vi "Side E.vi"(0 "Input Image":T7, 1 "Calibrated Image":T7, 5 "Ref ROI Parameters":T6={"Ref Line ROI Before Transformation"={"Global Rectangle"=[], "Contours"=[]}, "Ref ROI Search Direction"=2, "Ref ROI Edge Options"={"Edge Polarity"=2, "Kernel Size"=3, "Width"=3, "Minimum Edge Strength"=50.0, "Interpolation Type"=enum."Zero Order", "Data Processing Method"=enum."Average"}, "Ref ROI Line Options"={"Number of Lines"=1, "Type"=enum."Best Edge Rake", "Min. Score"=10.0, "Max. Score"=1000.0, "Orientation"=0.0, "Angle Range"=10.0, "Angle Tolerance"=10.0, "Step Size"=14, "Min. SNR (db)"=0.0, "Min. Points (%)"=25.0, "Hough Iterations"=5}, "Ref ROI Overlay"=FALSE, "Ref Rake Line Overlay 2"=FALSE, "Ref Edge/Point Overlay"=FALSE} {"Ref ROI Line Options"."Min. Points (%)" min=0.0 max=100.0; "Ref ROI Line Options"."Min. SNR (db)" min=0.0; "Ref ROI Line Options"."Max. Score" min=0.0 max=1024.0; "Ref ROI Line Options"."Min. Score" min=0.0 max=1024.0 step=1.0; "Ref ROI Edge Options"."Edge Polarity" items=["All Edges", "Rising Edges", "Falling Edges"]; "Ref ROI Edge Options"."Minimum Edge Strength" format="%.2f"; "Ref ROI Edge Options"."Width" step=2; "Ref ROI Edge Options"."Kernel Size" step=2; "Ref ROI Search Direction" items=["Left to Right", "Right to Left", "Top to Bottom", "Bottom to Top"]}, 7 "Measurement ROI Parameters":T3={"ROI 1 Before Transformation"={"Global Rectangle"=[], "Contours"=[]}, "ROI 1 Scan Direction"=0, "ROI 1 Edge Options"={"Edge Polarity"=0, "Kernel Size"=3, "Width"=3, "Minimum Edge Strength"=50.0, "Interpolation Type"=enum."Zero Order", "Data Processing Method"=enum."Average"}, "ROI 1Step Size"=3, "ROI 1 Process"=enum."Get First + Last Edge", "ROI 1 Overlay"=FALSE, "ROI 1 Rake Line Overlay"=FALSE, "ROI 1 Edge/Point Overlay"=FALSE} {"ROI 1 Edge Options"."Edge Polarity" items=["All Edges", "Rising Edges", "Falling Edges"]; "ROI 1 Edge Options"."Minimum Edge Strength" format="%.2f"; "ROI 1 Edge Options"."Width" step=2; "ROI 1 Edge Options"."Kernel Size" step=2; "ROI 1 Scan Direction" items=["Left To Right", "Right To Left", "Top To Bottom", "Bottom To Top"]}, 9 "AvgMinMax 2":enum16{"Average", "Max", "Min", "Max2"}(ring), 11 "error in (no error)":errorcluster, 12 "Center X &Y":cluster{"Center X":dbl, "Center Y":dbl}) -> (4 "Image Out":T7(plugin-control), 6 "output cluster":T8, 15 "error out":errorcluster)   [LabVIEW 2019, in "Algorithm.lvclass"]
doc: "The reference used to find the reference straight line. \nThen find middle point on this line.\nWith respect to this point decide measurement ROI.\nCalculate measurement using the IMAQ Rake3."
uses:
  FrameworkOverrides/Algorithm.lvclass
  <vilib>/vision/NI_Vision_Development_Module.lvlib
  <vilib>/vision/Measure.llb/Edge Polarity.ctl
  <vilib>/vision/Measure.llb/Edge Options.ctl
  <vilib>/vision/Measure.llb/Straight Edge Process.ctl
  <vilib>/vision/Measure.llb/Straight Edge Options.ctl
  <vilib>/vision/Image Controls.llb/IMAQ Image.ctl
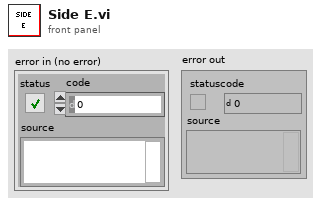
[diagram p1: front panel]
types:
  T1 = typedef "Edge Options.ctl" = cluster{"Edge Polarity":T2, "Kernel Size":u32, "Width":u32, "Minimum Edge Strength":sgl, "Interpolation Type":enum32{"Zero Order", "Bilinear", "Quadratic", "Cubic", "Bilinear Fixed"}, "Data Processing Method":enum32{"Average", "Median"}}
  T2 = typedef "Edge Polarity.ctl" = u32
  T3 = cluster{"ROI 1 Before Transformation":cluster{"Global Rectangle":i32[], "Contours":cluster{"ID":enum32{"External", "Internal"}, "Type":u32, "Coordinates":i32[]}[]}, "ROI 1 Scan Direction":u16, "ROI 1 Edge Options":T1, "ROI 1Step Size":u32, "ROI 1 Process":enum16{"Get First Edge", "Get First + Last Edge", "Get All Edges", "Get Best Edge"}, "ROI 1 Overlay":bool, "ROI 1 Rake Line Overlay":bool, "ROI 1 Edge/Point Overlay":bool}
  T4 = typedef "Straight Edge Options.ctl" = cluster{"Number of Lines":i32, "Type":T5, "Min. Score":dbl, "Max. Score":dbl, "Orientation":dbl, "Angle Range":dbl, "Angle Tolerance":dbl, "Step Size":u32, "Min. SNR (db)":dbl, "Min. Points (%)":dbl, "Hough Iterations":i32}
  T5 = typedef "Straight Edge Process.ctl" = enum32{"First Edge Rake", "Best Edge Rake", "Hough Edge Rake", "First Edge Projection", "Best Edge Projection"}
  T6 = cluster{"Ref Line ROI Before Transformation":cluster{"Global Rectangle":i32[], "Contours":cluster{"ID":enum32{"External", "Internal"}, "Type":u32, "Coordinates":i32[]}[]}, "Ref ROI Search Direction":u32, "Ref ROI Edge Options":T1, "Ref ROI Line Options":T4, "Ref ROI Overlay":bool, "Ref Rake Line Overlay 2":bool, "Ref Edge/Point Overlay":bool}
  T7 = typedef "IMAQ Image.ctl" = refnum<image>
  T8 = cluster{"E Side EMeasurement":sgl, "Points for Arrow Overlay":cluster{"X":sgl, "Y":sgl}[]}
  T9 = typedef "IMAQ Rectangle" = cluster{"Left":i32, "Top":i32, "Right":i32, "Bottom":i32, "Rotation":dbl}
  T10 = cluster{"Global Rectangle":i32[], "Contours":cluster{"ID":enum32{"External", "Internal"}, "Type":u32, "Coordinates":i32[]}[]}
  T11 = cluster{"ID":enum32{"External", "Internal"}, "Type":u32, "Coordinates":i32[]}[]
  T12 = cluster{"ID":enum32{"External", "Internal"}, "Type":u32, "Coordinates":i32[]}
  T13 = cluster{"Coordinates[0]":i32, "Coordinates[1]":i32, "Coordinates[2]":i32, "Coordinates[3]":i32, "Coordinates[4]":i32, "Coordinates[5]":i32, "Coordinates[6]":i32, "Coordinates[7]":i32, "Coordinates[8]":i32}
  T14 = typedef "ROI Descriptor" = cluster{"Global Rectangle":i32[], "Contours":cluster{"ID":enum32{"External", "Internal"}, "Type":u32, "Coordinates":i32[]}[]}
  T15 = cluster{"Point1 (Pixels)":cluster{"X":sgl, "Y":sgl}, "Point2 (Pixels)":cluster{"X":sgl, "Y":sgl}, "Point1 (Real-World)":cluster{"X":sgl, "Y":sgl}, "Point2 (Real-World)":cluster{"X":sgl, "Y":sgl}, "Angle (Pixel)":dbl, "Angle (Real-World)":dbl, "Score":dbl, "Straightness":dbl, "Average SNR (db)":dbl, "Calibration Valid":bool}[]
  T16 = typedef "Search Line.ctl" = cluster{"Start Point":cluster{"X":sgl, "Y":sgl}, "End Point":cluster{"X":sgl, "Y":sgl}, "Edge Info":T17[], "Edge Map":dbl[], "Calibration Valid":bool}
  T17 = typedef "Edge New.ctl" = cluster{"Location (Pixel)":cluster{"X":sgl, "Y":sgl}, "Location (Real-World)":cluster{"X":sgl, "Y":sgl}, "Distance (Pixel)":dbl, "Distance (Real-World)":dbl, "Strength":dbl, "Noise":dbl, "Rising?":bool}
  T18 = cluster{"Point1 (Pixels)":cluster{"X":sgl, "Y":sgl}, "Point2 (Pixels)":cluster{"X":sgl, "Y":sgl}, "Point1 (Real-World)":cluster{"X":sgl, "Y":sgl}, "Point2 (Real-World)":cluster{"X":sgl, "Y":sgl}, "Angle (Pixel)":dbl, "Angle (Real-World)":dbl, "Score":dbl, "Straightness":dbl, "Average SNR (db)":dbl, "Calibration Valid":bool}
  T19 = enum16{"Get First Edge", "Get First + Last Edge", "Get All Edges", "Get Best Edge"}
  T20 = cluster{"Location (Pixel)":cluster{"X":sgl, "Y":sgl}, "Location (Pixel)":cluster{"X":sgl, "Y":sgl}}
  T21 = cluster{"Start Point":cluster{"X":sgl, "Y":sgl}, "Location (Pixel)":cluster{"X":sgl, "Y":sgl}, "Location (Pixel)":cluster{"X":sgl, "Y":sgl}, "End Point":cluster{"X":sgl, "Y":sgl}}
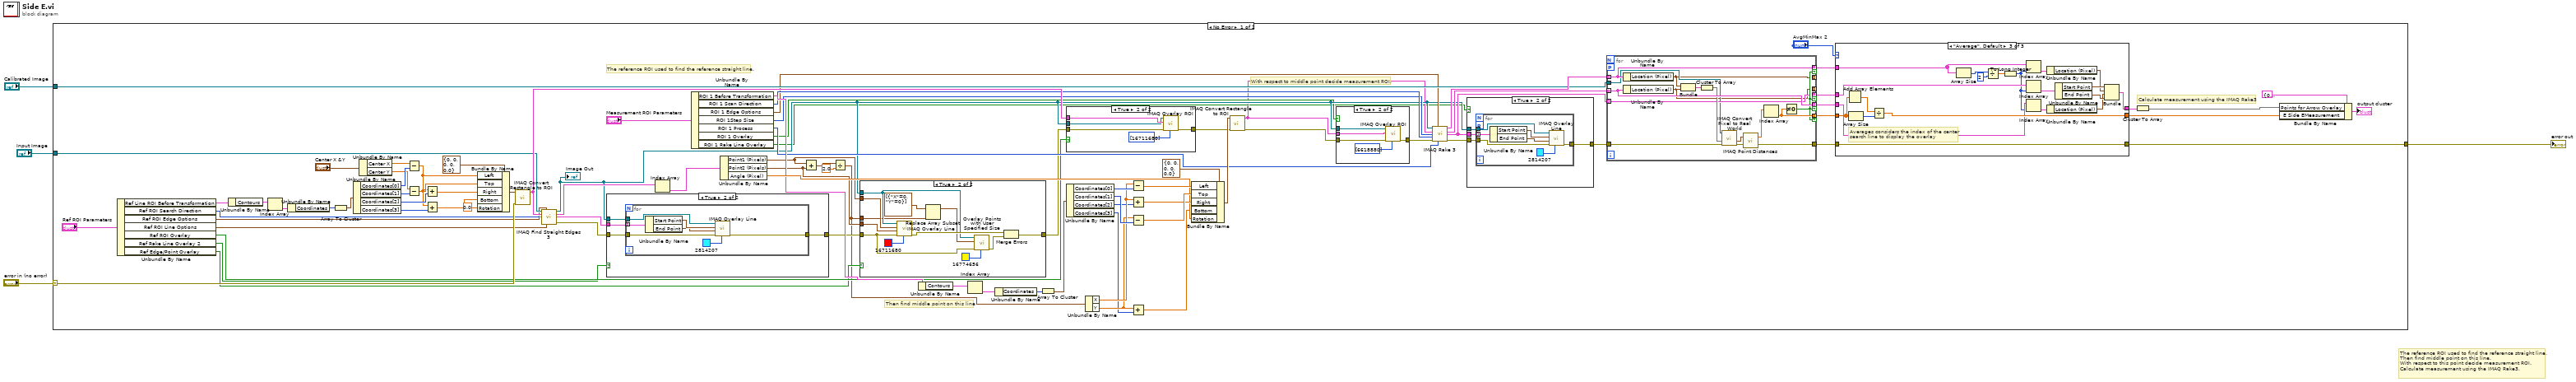
[diagram p0: block diagram]
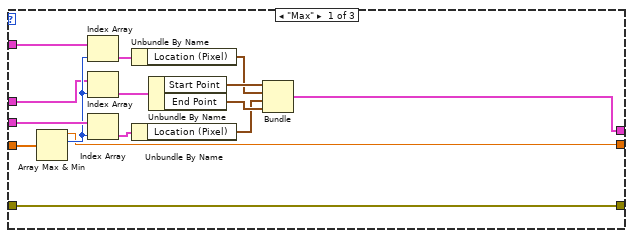
[diagram p7: hidden frame]
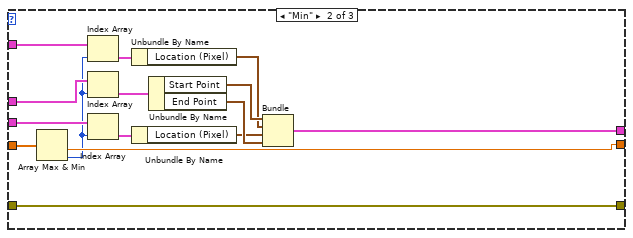
[diagram p8: hidden frame]
diagram:
  # "The reference ROI used to find the reference straight line. \nThen find middle point on this line.\nWith respect to this point decide measurement ROI.\nCalculate measurement using the IMAQ Rake3."
  n1 = case shown="No Error" "error in (no error)" {
    selector: "error in (no error)" -> [w47 w207]
    tunnel: [w34 w207] -> w4
    tunnel: "Input Image" -> [w39 _]
    tunnel: "Calibrated Image" -> [w37 _]
    frame No Error {
      # "Calculate measurement using the IMAQ Rake3"
      # "With respect to middle point decide measurement ROI."
      # "Then find middle point on this line"
      # "The reference ROI used to find the reference straight line."
      n2 = Unbundle By Name("Ref ROI Parameters") -> ("Ref Line ROI Before Transformation"=w32:T10, "Ref ROI Search Direction"=w30:u32, "Ref ROI Edge Options"=w31:T1, "Ref ROI Line Options"=w29:T4, "Ref ROI Overlay"=w22:bool, "Ref Rake Line Overlay 2"=w19:bool, "Ref Edge/Point Overlay"=w14:bool)
      n3 = Unbundle By Name(w32) -> ("Contours"=w81:T11)
      n4 = Index Array(array=w81) -> (element=w80:T12)  [unwired: 1 in]
      n5 = Unbundle By Name(w80) -> ("Coordinates"=w82:i32[])
      n6 = Array To Cluster(array=w82) -> (cluster=w83:T13)
      n7 = Unbundle By Name(w83) -> ("Coordinates[0]"=w84:i32, "Coordinates[1]"=w85:i32, "Coordinates[2]"=w86:i32, "Coordinates[3]"=w87:i32)
      n8 = Unbundle By Name("Center X &Y") -> ("Center X"=w71:dbl, "Center Y"=w73:dbl)
      n9 = Subtract(x=w71, y=w84) -> (x-y=w74:dbl)
      n10 = Subtract(x=w73, y=w85) -> (x-y=w76:dbl)
      n11 = Add(x=w74, y=w86) -> (x+y=w75:dbl)
      n12 = Add(x=w76, y=w87) -> (x+y=w77:dbl)
      n13 = Bundle By Name(cluster=T9 {"Left"=0, "Top"=0, "Right"=0, "Bottom"=0, "Rotation"=0.0} ("Rectangle"), "Left"=w74, "Top"=w76, "Right"=w75, "Bottom"=w77, "Rotation"=0.0 ("y")) -> (w79:T9)
      n14 = call "IMAQ Convert Rectangle to ROI"("error in (no error)"=w47, "Rectangle"=w79) -> ("ROI Descriptor"=w46:T14)  [unwired: 7 in, 1 out]
      n15 = call "IMAQ Find Straight Edges 3"("Image"=w39, "Edge Options"=w31, "ROI Descriptor"=w46, "Search Direction"=w30, "Line Options"=w29) -> ("Image (duplicate)"=w11:T7, "Straight Edges"=w92:T15, "Search Lines Information"=w38:T16[], "error out"=w20:errorcluster)  [unwired: 6 in, 1 out]
      "Image Out" <- w11
      n16 = case shown="True" w19 {
        tunnel: w38 -> [_ w128]
        tunnel: w11 -> [_ w127]
        tunnel: w20 -> [w124 w126]
        tunnel: [w124 w125] -> w16
        frame False {
        }
        frame True {
          n17 = for {
            tunnel: w128 -> [w135] mode=indexing
            tunnel: w127 -> [w132]
            tunnel: w126 -> [w130]
            tunnel: [w129] -> w125
            n18 = Unbundle By Name(w135) -> ("Start Point"=w134:cluster{"X":sgl, "Y":sgl}, "End Point"=w133:cluster{"X":sgl, "Y":sgl})
            n19 = call "IMAQ Overlay Line"("Color"=u32 2814207, "error in (no error)"=w130, "End Point"=w133, "Start Point"=w134, "Image"=w132) -> ("error out"=w129:errorcluster)  [unwired: 5 in, 1 out]
          }
        }
      }
      n20 = Index Array(array=w92) -> (element=w68:T18)  [unwired: 1 in]
      n21 = Unbundle By Name("Measurement ROI Parameters") -> ("ROI 1 Before Transformation"=w27:T10, "ROI 1 Scan Direction"=w26:u16, "ROI 1 Edge Options"=w24:T1, "ROI 1Step Size"=w25:u32, "ROI 1 Process"=w23:T19, "ROI 1 Overlay"=w9:bool, "ROI 1 Rake Line Overlay"=w5:bool)
      n22 = Unbundle By Name(w68) -> ("Point1 (Pixels)"=w17:cluster{"X":sgl, "Y":sgl}, "Point2 (Pixels)"=w18:cluster{"X":sgl, "Y":sgl}, "Angle (Pixel)"=w45:dbl)
      n23 = Add(x=w17, y=w18) -> (x+y=w69:cluster{"X":sgl, "Y":sgl})
      n24 = Divide(x=w69, y=2.0) -> (x/y=w13:cluster{"X":dbl, "Y":dbl})
      n25 = case shown="True" w14 {
        tunnel: w18 -> [_ w123]
        tunnel: w17 -> [_ w122]
        tunnel: w11 -> [_ w118]
        tunnel: w16 -> [w111 w120]
        tunnel: [w111 w114] -> w15
        tunnel: w13 -> [_ w116]
        frame False {
        }
        frame True {
          n26 = call "IMAQ Overlay Line"("Color"=u32 16711680, "error in (no error)"=w120, "End Point"=w123, "Start Point"=w122, "Image"=w118) -> ("error out"=w121:errorcluster)  [unwired: 5 in, 1 out]
          n27 = Replace Array Subset(array=cluster{"X":i32, "Y":i32}[] [{"X"=0, "Y"=0}] ("Points"), new element=w116) -> (w115:cluster{"X":i32, "Y":i32}[])  [unwired: 1 in]
          n28 = call "Overlay Points with User Specified Size.vi"("Color"=u32 16774656, "error in"=w120, "Points"=w115, "Image In"=w118) -> ("error out"=w119:errorcluster)  [unwired: 6 in, 1 out]
          n29 = Merge Errors(w121, w119) -> (w114:errorcluster)
        }
      }
      n30 = Unbundle By Name(w27) -> ("Contours"=w88:T11)
      n31 = Index Array(array=w88) -> (element=w89:T12)  [unwired: 1 in]
      n32 = Unbundle By Name(w89) -> ("Coordinates"=w91:i32[])
      n33 = Array To Cluster(array=w91) -> (cluster=w90:T13)
      n34 = case shown="True" w22 {
        tunnel: w46 -> [_ w141]
        tunnel: w11 -> [_ w139]
        tunnel: [w136 w138] -> w21
        tunnel: w15 -> [w136 w137]
        frame False {
        }
        frame True {
          n35 = call "IMAQ Overlay ROI"("Colors (Green)"=u32[] [16711680], "error in (no error)"=w137, "ROI Descriptor"=w141, "Image"=w139) -> ("error out"=w138:errorcluster)  [unwired: 6 in, 1 out]
        }
      }
      n36 = Unbundle By Name(w90) -> ("Coordinates[0]"=w67:i32, "Coordinates[1]"=w65:i32, "Coordinates[2]"=w62:i32, "Coordinates[3]"=w59:i32)
      n37 = Unbundle By Name(w13) -> ("X"=w63:dbl, "Y"=w60:dbl)
      n38 = Subtract(x=w63, y=w67) -> (x-y=w66:dbl)
      n39 = Add(x=w63, y=w62) -> (x+y=w61:dbl)
      n40 = Subtract(x=w60, y=w65) -> (x-y=w64:dbl)
      n41 = Add(x=w60, y=w59) -> (x+y=w41:dbl)
      n42 = Bundle By Name(cluster=T9 {"Left"=0, "Top"=0, "Right"=0, "Bottom"=0, "Rotation"=0.0} ("Rectangle"), "Left"=w66, "Top"=w64, "Right"=w61, "Bottom"=w41, "Rotation"=w45) -> (w57:T9)
      n43 = call "IMAQ Convert Rectangle to ROI"("error in (no error)"=w21, "Rectangle"=w57) -> ("error out"=w12:errorcluster, "ROI Descriptor"=w6:T14)  [unwired: 7 in]
      n44 = case shown="True" w9 {
        tunnel: w12 -> [w105 w108]
        tunnel: w11 -> [_ w110]
        tunnel: [w105 w107] -> w10
        tunnel: w6 -> [_ w106]
        frame False {
        }
        frame True {
          n45 = call "IMAQ Overlay ROI"("Colors (Green)"=u32[] [6618880], "error in (no error)"=w108, "ROI Descriptor"=w106, "Image"=w110) -> ("error out"=w107:errorcluster)  [unwired: 6 in, 1 out]
        }
      }
      n46 = call "IMAQ Rake 3"("Image"=w11, "Edge Options"=w24, "ROI Descriptor"=w6, "Step Size"=w25, "Scan Direction"=w26, "error in (no error)"=w10, "Process"=w23) -> ("First Edges"=w43:T17[], "Last Edges"=w56:T17[], "Search Lines"=w42:T16[], "error out"=w8:errorcluster)  [unwired: 5 in]
      n47 = case shown="True" w5 {
        tunnel: w42 -> [_ w97]
        tunnel: w11 -> [_ w96]
        tunnel: w8 -> [w93 w95]
        tunnel: [w93 w94] -> w7
        frame False {
        }
        frame True {
          n48 = for {
            tunnel: w97 -> [w104] mode=indexing
            tunnel: w96 -> [w101]
            tunnel: w95 -> [w99]
            tunnel: [w98] -> w94
            workers-P: _ -> [_]
            n49 = Unbundle By Name(w104) -> ("Start Point"=w103:cluster{"X":sgl, "Y":sgl}, "End Point"=w102:cluster{"X":sgl, "Y":sgl})
            n50 = call "IMAQ Overlay Line"("Color"=u32 2814207, "error in (no error)"=w99, "End Point"=w102, "Start Point"=w103, "Image"=w101) -> ("error out"=w98:errorcluster)  [unwired: 5 in, 1 out]
          }
        }
      }
      n51 = for {
        tunnel: w43 -> [w201] mode=indexing
        tunnel: w56 -> [w202] mode=indexing
        tunnel: w42 -> [w197] mode=indexing
        tunnel: [w204] -> w51 mode=indexing if=w200
        tunnel: w7 -> [w195]
        tunnel: [w205] -> w35
        tunnel: [w197] -> w52 mode=indexing if=w200
        tunnel: [w202] -> w54 mode=indexing if=w200
        tunnel: [w201] -> w53 mode=indexing if=w200
        tunnel: w37 -> [w196]
        tunnel: [w193] -> _ mode=indexing
        tunnel: [w192] -> _ mode=indexing
        workers-P: _ -> [_]
        n52 = Unbundle By Name(w201) -> ("Location (Pixel)"=w192:cluster{"X":sgl, "Y":sgl})
        n53 = Unbundle By Name(w202) -> ("Location (Pixel)"=w193:cluster{"X":sgl, "Y":sgl})
        n54 = Bundle("Location (Pixel)"=w192, "Location (Pixel)"=w193) -> (w203:T20)  [unwired: 1 in]
        n55 = Cluster To Array(cluster=w203) -> (array=w199:cluster{"X":sgl, "Y":sgl}[])
        n56 = call "IMAQ Convert Pixel to Real World"("error in (no error)"=w195, "Array of Pixel Coordinates"=w199, "Calibrated Image"=w196) -> ("error out"=w194:errorcluster, "Array of Real World Coordinates"=w198:cluster{"X":sgl, "Y":sgl}[])  [unwired: 3 in, 4 out]
        n57 = call "IMAQ Point Distances"("Points"=w198, "error in (no error)"=w194) -> ("Distances"=w206:sgl[], "error out"=w205:errorcluster)  [unwired: 3 in]
        n58 = Index Array(array=w206) -> (element=w204:sgl)  [unwired: 1 in]
        n59 = Not Equal To 0?(x=w204) -> (x != 0?=w200:bool)
      }
      n60 = case shown="\"Average\", Default" "AvgMinMax 2" {
        tunnel: [w143 w170 w191] -> w44
        tunnel: w51 -> [w156 w171 w178]
        tunnel: w53 -> [w155 w164 w184]
        tunnel: w54 -> [w153 w166 w186]
        tunnel: w52 -> [w149 w165 w185]
        tunnel: [w148 w162 w187] -> w55
        tunnel: w35 -> [w142 w157 w172]
        tunnel: [w142 w157 w172] -> w34
        frame "Max" {
          n61 = Array Max & Min(array=w156) -> (max value=w143:sgl, max index (indices)=w152:i32)  [unwired: 2 out]
          n62 = Index Array(array=w155, index=w152) -> (element=w154:T17)
          n63 = Index Array(array=w149, index=w152) -> (element=w150:T16)
          n64 = Index Array(array=w153, index=w152) -> (element=w151:T17)
          n65 = Unbundle By Name(w154) -> ("Location (Pixel)"=w145:cluster{"X":sgl, "Y":sgl})
          n66 = Unbundle By Name(w151) -> ("Location (Pixel)"=w144:cluster{"X":sgl, "Y":sgl})
          n67 = Unbundle By Name(w150) -> ("Start Point"=w147:cluster{"X":sgl, "Y":sgl}, "End Point"=w146:cluster{"X":sgl, "Y":sgl})
          n68 = Bundle("Start Point"=w147, "Location (Pixel)"=w145, "Location (Pixel)"=w144, "End Point"=w146) -> (w148:T21)  [unwired: 1 in]
        }
        frame "Min" {
          n69 = Array Max & Min(array=w171) -> (min value=w170:sgl, min index (indices)=w163:i32)  [unwired: 2 out]
          n70 = Index Array(array=w164, index=w163) -> (element=w167:T17)
          n71 = Index Array(array=w165, index=w163) -> (element=w169:T16)
          n72 = Index Array(array=w166, index=w163) -> (element=w168:T17)
          n73 = Unbundle By Name(w167) -> ("Location (Pixel)"=w159:cluster{"X":sgl, "Y":sgl})
          n74 = Unbundle By Name(w168) -> ("Location (Pixel)"=w158:cluster{"X":sgl, "Y":sgl})
          n75 = Unbundle By Name(w169) -> ("Start Point"=w161:cluster{"X":sgl, "Y":sgl}, "End Point"=w160:cluster{"X":sgl, "Y":sgl})
          n76 = Bundle("Start Point"=w161, "Location (Pixel)"=w159, "Location (Pixel)"=w158, "End Point"=w160) -> (w162:T21)  [unwired: 1 in]
        }
        frame "Average", Default {
          # "Averages considers the index of the center \nsearch line to display the overlay"
          n77 = Add Array Elements(numeric array=w178) -> (sum=w176:sgl)
          n78 = Array Size(array=w178) -> (size(s)=w177:i32)
          n79 = Divide(x=w176, y=w177) -> (x/y=w191:sgl)
          n80 = Array Size(array=w184) -> (size(s)=w175:i32)
          n81 = Divide(x=w175, y=2) -> (x/y=w183:dbl)
          n82 = To Long Integer(number=w183) -> (32bit integer=w174:i32)
          n83 = Index Array(array=w184, index=w174) -> (element=w190:T17)
          n84 = Index Array(array=w185, index=w174) -> (element=w188:T16)
          n85 = Index Array(array=w186, index=w174) -> (element=w189:T17)
          n86 = Unbundle By Name(w190) -> ("Location (Pixel)"=w180:cluster{"X":sgl, "Y":sgl})
          n87 = Unbundle By Name(w189) -> ("Location (Pixel)"=w179:cluster{"X":sgl, "Y":sgl})
          n88 = Unbundle By Name(w188) -> ("Start Point"=w182:cluster{"X":sgl, "Y":sgl}, "End Point"=w181:cluster{"X":sgl, "Y":sgl})
          n89 = Bundle("Start Point"=w182, "Location (Pixel)"=w180, "Location (Pixel)"=w179, "End Point"=w181) -> (w187:T21)  [unwired: 1 in]
        }
      }
      n90 = Cluster To Array(cluster=w55) -> (array=w50:cluster{"X":sgl, "Y":sgl}[])
      n91 = Bundle By Name(cluster=T8 {"E Side EMeasurement"=0.0, "Points for Arrow Overlay"=[]}, "Points for Arrow Overlay"=w50, "E Side EMeasurement"=w44) -> (→"output cluster":T8)
    }
    frame Error {
    }
  }
  "error out" <- w4
